vi "Launch Handler.vi"(4 "UUID":string, 6 "data model":refnum<class "Device Data Model.lvclass">, 8 "error in (no error)":errorcluster, 9 "transmission data unit":refnum<class "Transmission Data Unit.lvclass">, 10 "connection reference":refnum<data-value>, 11 "TCP slave":refnum<class "TCP Slave.lvclass">) -> (0 "error out":errorcluster)   [LabVIEW 2020, in "SubVIs.lvlib" / "TCP Slave.lvclass"]
doc: "Asynchronously launches a connection handler."
uses:
  <vilib>/Modbus/subvis/Protocol/TCP/TCP Slave/TCP Slave.lvclass
  <vilib>/Modbus/subvis/Transmission Data Unit (ADU)/Transmission Data Unit/Transmission Data Unit.lvclass
  <vilib>/Modbus/subvis/Data and Functions/Device Data Model/Device Data Model.lvclass
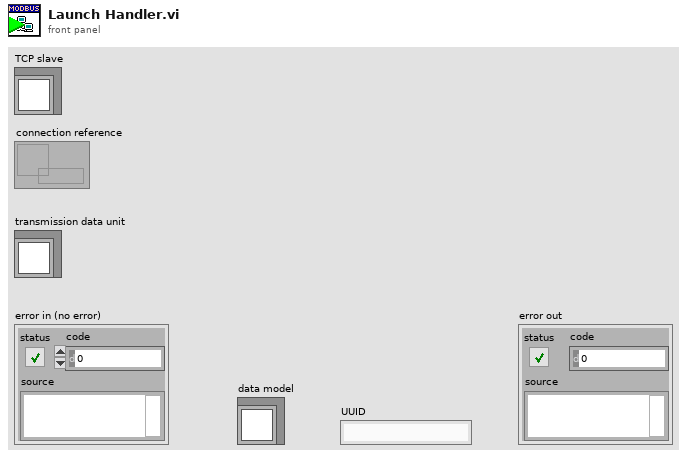
[diagram p1: front panel]
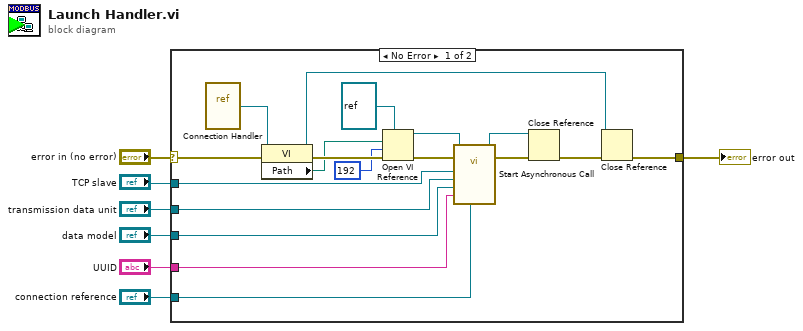
[diagram p0: block diagram]
diagram:
  n1 = case shown="No Error" "error in (no error)" {
    selector: "error in (no error)" -> [w12 w26]
    tunnel: "transmission data unit" -> [w25 _]
    tunnel: "UUID" -> [w17 _]
    tunnel: "TCP slave" -> [w16 _]
    tunnel: "data model" -> [w15 _]
    tunnel: "connection reference" -> [w14 _]
    tunnel: [w10 w26] -> w2
    frame No Error {
      n2 = vi-ref <vilib>:"Connection Handler.vi"() -> (w24:refnum<vi>)
      n3 = property class="VI"(reference=w24, error in=w12) -> (reference out=w8:refnum<vi>, error out=w23:errorcluster, "Path"=w21:path)
      n4 = Open VI Reference(type specifier VI Refnum (for type only)=refnum<vi> refnum, vi path=w21, options=192 ("x .or. y?"), error in (no error)=w23) -> (vi reference=w18:refnum<vi>, error out=w19:errorcluster)  [unwired: 2 in]
      n5 = call-by-ref "Start Asynchronous Call"(reference=w18, error in=w19, "connection reference"=w14, "UUID"=w17, "Data Model"=w15, "transmission data unit"=w25, "TCP slave"=w16) -> (reference out=w9:refnum<vi>, error out=w13:errorcluster)  [unwired: 7 in]
      n6 = Close Reference(reference=w9, error in (no error)=w13) -> (error out=w11:errorcluster)
      n7 = Close Reference(reference=w8, error in (no error)=w11) -> (error out=w10:errorcluster)
    }
    frame Error {
    }
  }
  "error out" <- w2
